vi "LVClass_HasoSlopes ctor from copy.vi"(0 "HasoSlopes (const)":refnum<class "HasoSlopes.lvclass">, 5 "HasoSlopes ToCopy":refnum<class "HasoSlopes.lvclass">, 11 "error in (no error)":errorcluster) -> (4 "HasoSlopes (new)":refnum<class "HasoSlopes.lvclass">, 6 "HasoSlopes ToCopy (dup)":refnum<class "HasoSlopes.lvclass">, 15 "error out":errorcluster)   [LabVIEW 2020, in "HasoSlopes.lvclass"]
doc: "HasoSlopes constructor from copy.\n\n--------------------------------------------------------------------------------\n\n<B>HasoSlopesIn </B> : Constant Pointer to HasoSlopes object.\n<B>HasoSlopesOut </B> : Constant Pointer to HasoSlopes object.\n<B>HasoSlopes_src </B> : Pointer to HasoSlopes object to copy.\n<B>ErrorIn </B> : Error\n<B>ErrorOut </B> : Error\n\n--------------------------------------------------------------------------------"
uses:
  HasoSlopes.lvclass
  Handle creation.ctl
  HasoSlopes.lvclass/HasoSlopes.ctl
  LVClass_HasoSlopes Read HasoSlopes _ property.vi
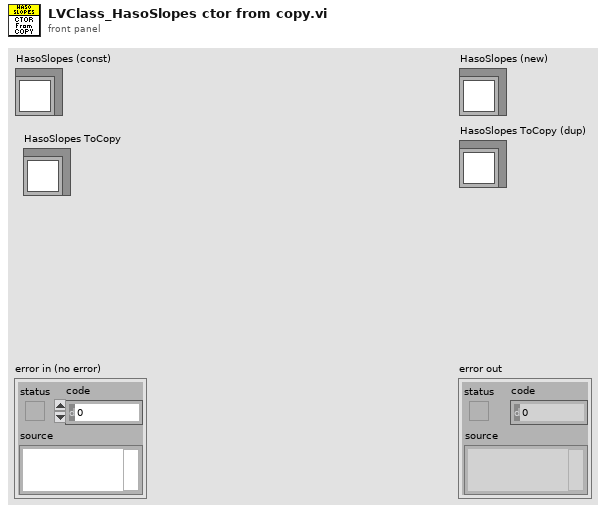
[diagram p1: front panel]
types:
  T1 = typedef "Handle creation.ctl" = enum16{"By ctor", "By write function"}
  T2 = typedef "ClassID.ctl" = i64
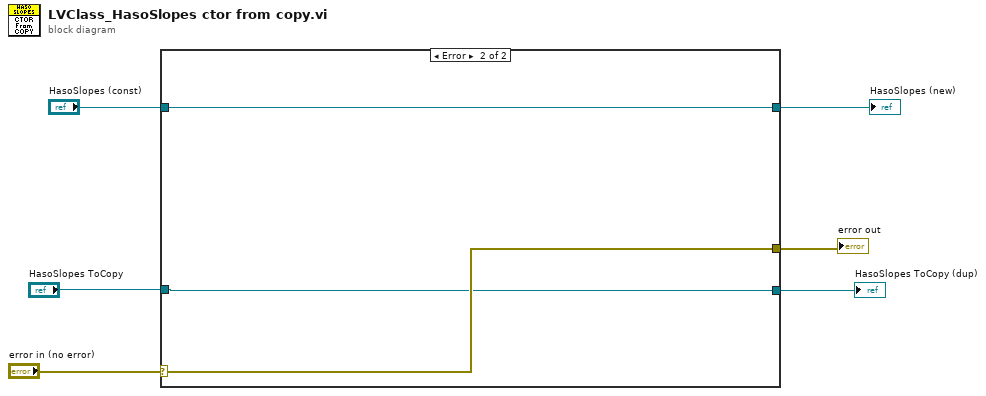
[diagram p0: block diagram]
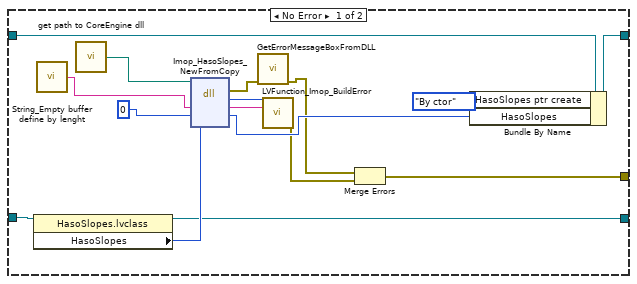
[diagram p2: hidden frame]
diagram:
  n1 = case shown="Error" "error in (no error)" {
    selector: "error in (no error)" -> [_ w25]
    tunnel: [w8 w25] -> w3
    tunnel: [w22 w24] -> w4
    tunnel: "HasoSlopes (const)" -> [w13 w24]
    tunnel: "HasoSlopes ToCopy" -> [w12 w23]
    tunnel: [w7 w23] -> w1
    frame No Error {
      n2 = property class="HasoSlopes.lvclass"(reference=w12) -> (reference out=w7:refnum<class "HasoSlopes.lvclass">, "HasoSlopes"=w11:T2)  [unwired: 1 in, 1 out]
      n3 = call "String_Empty buffer define by lenght.vi"() -> ("Empty buffer"=w20:string)  [unwired: 1 in]
      n4 = call "get path to CoreEngine dll.vi"() -> ("path to wavekit library"=w21:path)  [unwired: 14 in, 1 out]
      n5 = dll-call lib="D:/soft/HASO_v3/SVN_trunk/ImOpCoreEngine4_LV2011/DLLs/c_interface_vc100.dll" fn="Imop_HasoSlopes_NewFromCopy"(path in=w21, "message"=w20, "objet"=0, "HasoSlopesCopy"=w11) -> (error out=w18:errorcluster, "return type"=w17:i32, "message"=w16:string, "objet"=w15:i64)  [unwired: 3 in, 1 out]
      n6 = call "GetErrorMessageBoxFromDLL.vi"("error IN"=w18) -> ("error OUT"=w10:errorcluster)  [unwired: 10 in]
      n7 = call "LVFunction_Imop_BuildError.vi"("code"=w17, "String to Prepend to source (\"\")"=w16) -> ("error out"=w9:errorcluster)  [unwired: 13 in]
      n8 = Merge Errors(w10, w9) -> (w8:errorcluster)
      n9 = Bundle By Name(cluster=w13, "HasoSlopes ptr create"=Handle_creation."By ctor", "HasoSlopes"=w15) -> (w22:refnum<class "HasoSlopes.lvclass">)
    }
    frame Error {
    }
  }
  "error out" <- w3
  "HasoSlopes (new)" <- w4
  "HasoSlopes ToCopy (dup)" <- w1
